vi "exit application if runtime.vi"(8 "error in":errorcluster) -> (0 "error out":errorcluster)   [LabVIEW 2023, in "Reusable Library.lvlib"]
uses:
  Reusable Library.lvlib
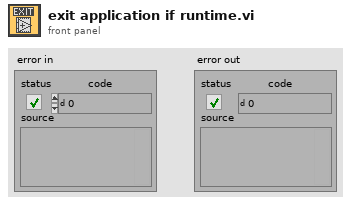
[diagram p1: front panel]
types:
  T1 = enum32{"invalid app kind", "Development System", "Run Time System", "Student Edition", "Embedded LabVIEW", "Evaluation", "Custom"}
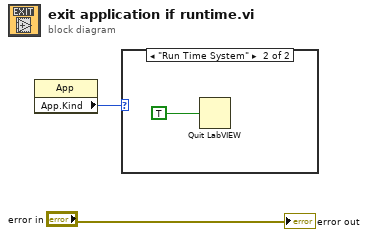
[diagram p0: block diagram]
diagram:
  n1 = property class="App"() -> ("App.Kind"=w1:T1)  [unwired: 2 in, 2 out]
  n2 = case shown="\"Run Time System\"" w1 {
    frame Default {
    }
    frame "Run Time System" {
      n3 = Quit LabVIEW(quit? (T)=TRUE) -> ()
    }
  }
  "error out" <- "error in"
